vi "BackgroundJump.vi"(8 "Current Index":dbl, 9 "Condition":dbl, 10 "isCalled":bool, 11 "Return Index":dbl) -> (1 "Done":bool, 3 "New Index":dbl)   [LabVIEW 2013]
uses:
  Robot Global Data.vi
  Common Code/Change Detect Boolean.vi
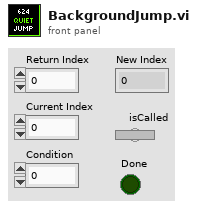
[diagram p1: front panel]
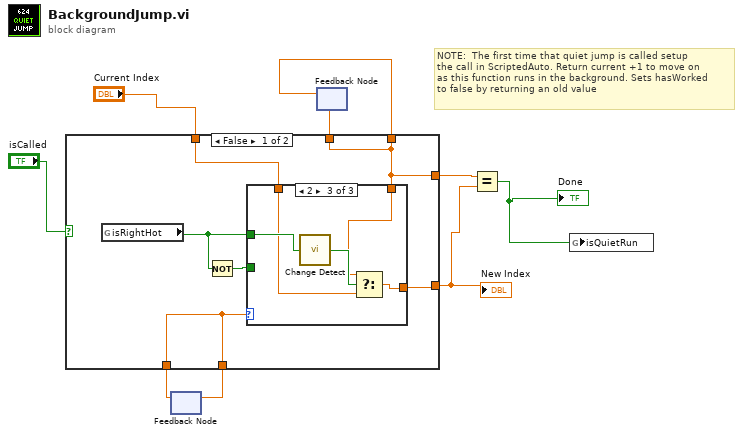
[diagram p0: block diagram]
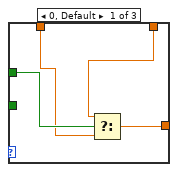
[diagram p2: hidden frame]
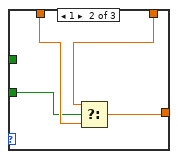
[diagram p3: hidden frame]
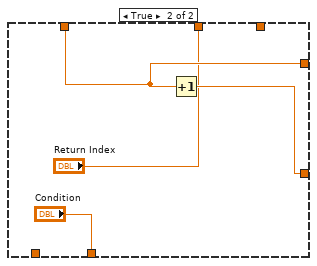
[diagram p4: hidden frame]
diagram:
  # "NOTE:  The first time that quiet jump is called setup \nthe call in ScriptedAuto. Return current +1 to move on \nas this function runs in the background. Sets hasWorked\nto false by returning an old value"
  n1 = feedback #1() -> (w2:dbl)  [unwired: 1 in]
  n2 = feedback #2() -> (w4:dbl)  [unwired: 1 in]
  n3 = case shown="False" "isCalled" {
    tunnel: [w13 w32] -> w8
    tunnel: "Current Index" -> [w11 w31]
    tunnel: [w10 w31] -> w7
    tunnel: w4 -> [w10 _]
    tunnel: [w10 "Return Index"] -> w5
    tunnel: [w12 "Condition"] -> w3
    tunnel: w2 -> [w12 _]
    frame False {
      n4 = global read "Robot Global Data.vi" "isRightHot"() -> (w15:bool)
      n5 = Not(x=w15) -> (.not. x?=w14:bool)
      n6 = case shown="2" w12 {
        tunnel: w11 -> [w17 w22 w24]
        tunnel: w10 -> [w16 w20 w26]
        tunnel: [w19 w23 w25] -> w13
        tunnel: w15 -> [w18 _ w28]
        tunnel: w14 -> [_ w21 _]
        frame 0, Default {
          n7 = Select(t=w16, s=w18, f=w17) -> (s? t:f=w19:dbl)
        }
        frame 1 {
          n8 = Select(t=w20, s=w21, f=w22) -> (s? t:f=w23:dbl)
        }
        frame 2 {
          n9 = call-poly "Change Detect.vi"("In"=w28) -> ("Changed?"=w27:bool)
          n10 = Select(t=w26, s=w27, f=w24) -> (s? t:f=w25:dbl)
        }
      }
    }
    frame True {
      n11 = Increment(x=w31) -> (x+1=w32:dbl)
    }
  }
  "New Index" <- w8
  n12 = feedback-in #1(w3) -> ()
  n13 = feedback-in #2(w5) -> ()
  n14 = Equal?(x=w7, y=w8) -> (x = y?=w6:bool)
  "Done" <- w6
  n15 = global write "Robot Global Data.vi" "isQuietRun"(w6) -> ()
